vi "ModifyTheValue.vi"(5 "property name":string, 7 "physical channel name":string, 8 "error in (no error)":errorcluster, 9 "Physical Channel Index Cluster":T1, 11 "Data":T2) -> (0 "error out":errorcluster, 2 "Physical Channel Index Cluster Out":T1, 3 "JSON Text Out":string)   [LabVIEW 2018]
uses:
  Ctrl/Data.ctl
  Ctrl/Caps.ctl
  Ctrl/Property.ctl
  Ctrl/PhysicalChannel.ctl
  Ctrl/Register.ctl
  Ctrl/Bitfield.ctl
  Ctrl/Scale.ctl
  Ctrl/ScaleType.ctl
  Ctrl/Enum.ctl
  Ctrl/EnumValue.ctl
  5d60f35e-cdab-4e3f-840e-4fbea60790d1.vi
  29d1ceb7-c941-4ae0-afee-51e252afae0f.vi
  d85de88c-8482-46f7-b9d0-abfa45f3a045.vi
  1afada16-43bf-44c8-a6ff-f358297126fe.vi
  df0b0e95-b0f6-4fc3-aeb6-1b22980748d9.vi
  ef347f2e-25c4-456b-8f90-f769631818f0.vi
  48839aac-ef3d-4912-a59c-d226e3977f89.vi
  0d674d4d-9f77-479f-94dc-be3b3816c1ec.vi
  5f0e6cbb-7cc1-45ab-b940-981c8c673de9.vi
  23bd61ce-0b3e-4435-9956-657a3c4ab8a9.vi
  1678344b-5bca-4df5-9ec5-619e6fe0b93b.vi
  e57232c7-e2d1-4d73-8c4d-58346bc82039.vi
  0e2d7ef8-d2e0-4754-b94e-53af8bd3d5fc.vi
  994b2aef-debc-40fb-8bd7-3405b5177060.vi
  ea1eb992-5890-4c98-ba09-5e0d2d65d542.vi
  <vilib>/JDP Science/JSONtext/String Subset.vi
  <vilib>/JDP Science/JSONtext/Parsing/Parse Full Path or Item Name.vi
  <vilib>/JDP Science/JSONtext/Offset/Find Item Locations by Path.vi
  <vilib>/JDP Science/JSONtext/JSON text to Variant.vi
  <vilib>/JDP Science/JSONtext/Variant to JSON Text.vi
  <vilib>/Utility/Data Type/NI_Data Type.lvlib
  <vilib>/JDP Science/JSONtext/JSONtext.lvlib
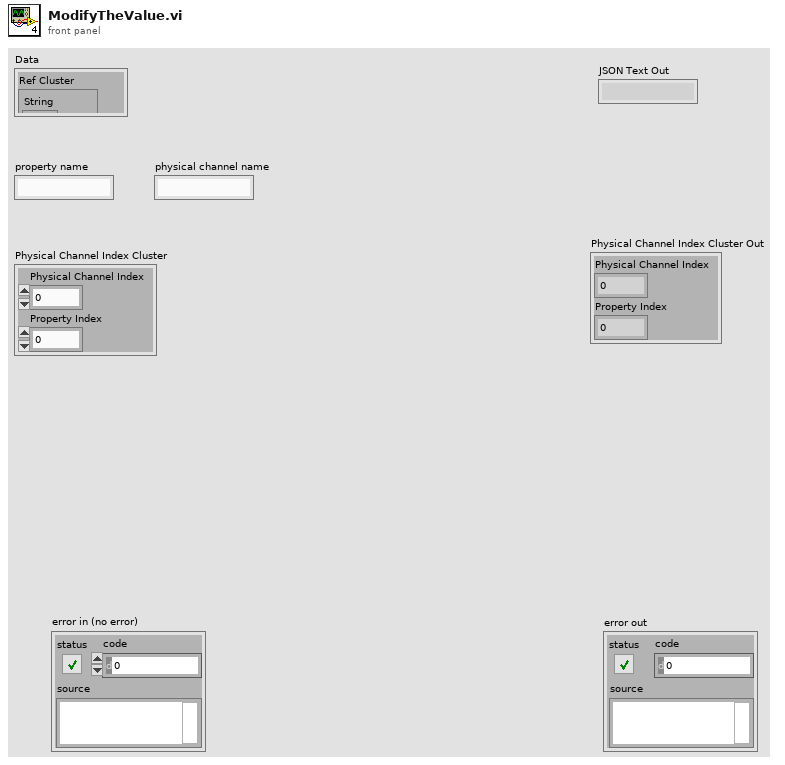
[diagram p1: front panel]
types:
  T1 = cluster{"Physical Channel Index":i32, "Property Index":i32}
  T2 = typedef "Data.ctl" = cluster{"Ref Cluster":cluster{"String":refnum<vi>, "U8":refnum<vi>, "I8":refnum<vi>, "U32":refnum<vi>, "I32":refnum<vi>, "U64":refnum<vi>, "I64":refnum<vi>, "Ring":refnum<vi>, "DBL":refnum<vi>, "Add":refnum<vi>, "Remove":refnum<vi>, "Property tree":refnum<vi>, "confirm":refnum<vi>}, "JSON Text":string, "Original JSON Text":string, "Caps":T3, "SLSC Output Tree":cluster{"Left Cell String":string, "Child Text":string[], "Child Tag":string, "Item Indent":i32, "Child Only?":bool, "Glyph Index":i32, "offline value":variant}[], "Ref Index and Control Type":cluster{"index":i32, "Datatype":string}, "Selected Type and name":cluster{"Selected Type":enum16{"Property", "Physical Channel", "Other"}, "Selected Property Name":string}, "Update whole Tree?":bool}
  T3 = typedef "Caps.ctl" = cluster{"properties":T4[], "physical channels":T5[], "registers":T6[], "scales":T8[], "enums":T10[], "productName":string}
  T4 = typedef "Property.ctl" = cluster{"name":string, "bitfield":string, "value":variant, "dataType":string, "min":variant, "max":variant, "scale":string, "access":string}
  T5 = typedef "PhysicalChannel.ctl" = cluster{"name":string, "properties":T4[]}
  T6 = typedef "Register.ctl" = cluster{"name":string, "address":i32, "size":i32, "bitfields":T7[], "initialValue":variant, "connectedProperties":string[]}
  T7 = typedef "Bitfield.ctl" = cluster{"name":string, "offset":i32, "size":i32, "signed":bool}
  T8 = typedef "Scale.ctl" = cluster{"name":string, "type":T9, "params":variant}
  T9 = typedef "ScaleType.ctl" = enum16{"NoScale", "Table", "Polynomial", "Linear"}
  T10 = typedef "Enum.ctl" = cluster{"name":string, "values":T11[]}
  T11 = typedef "EnumValue.ctl" = cluster{"name":string, "value":i32}
  T12 = typedef "NI_Data Type.lvlib/Data Type.ctl" = enum8{"Invalid Type", "Void", "I8", "I16", "I32", "I64", "U8", "U16", "U32", "U64", "Single Float", "Double Float", "Extended Float", "Single Complex", "Double Complex", "Extended Complex", "Enum U8", "Enum U16", "Enum U32", "Enum U64", "Single Float With Unit", "Double Float With Unit", "Extended Float With Unit", "Single Complex with Unit", "Double Complex with Unit", "Extended Complex with Unit", "Boolean", "String", "Path", "Picture", "Tag", "Array", "Cluster", "Variant", "LV Variant", "Waveform", "Timestamp", "Digital Waveform", "Digital Data", "ExpressData", "Refnum", "External Data", "VI", "Poly VI", "LabVIEW Class Instance", "Fixed Point"}
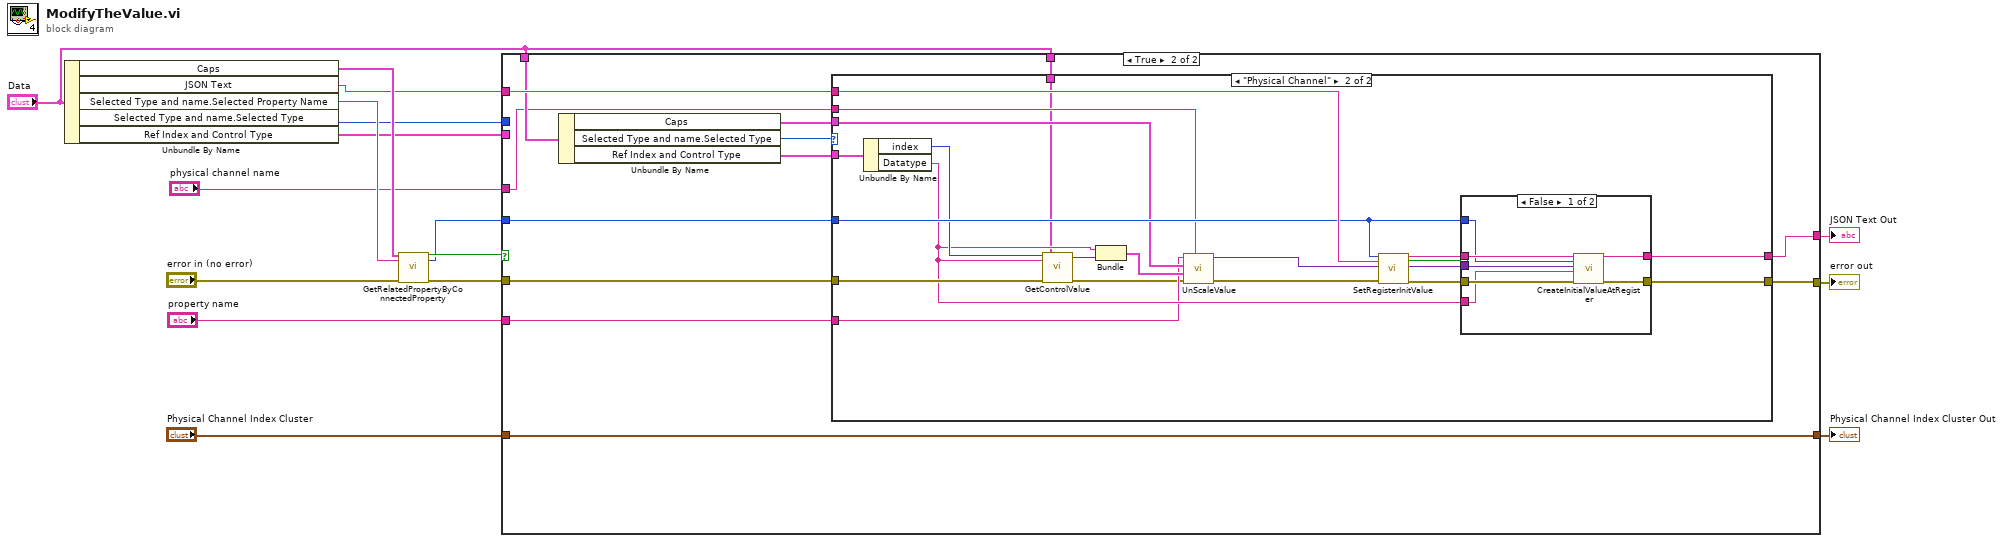
[diagram p0: block diagram]
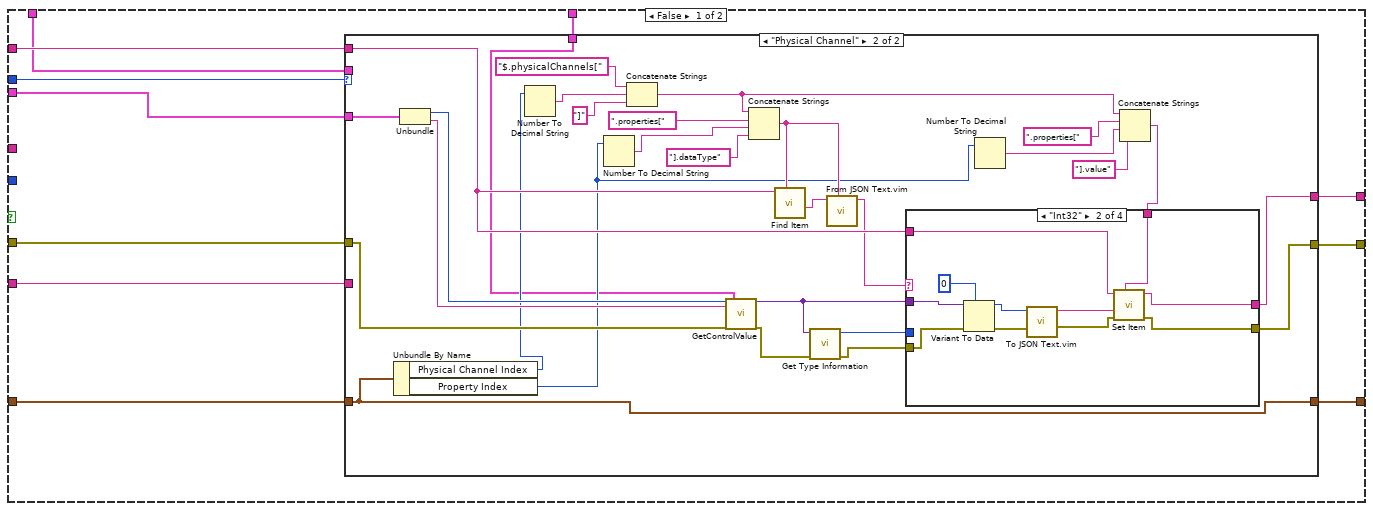
[diagram p2: hidden frame]
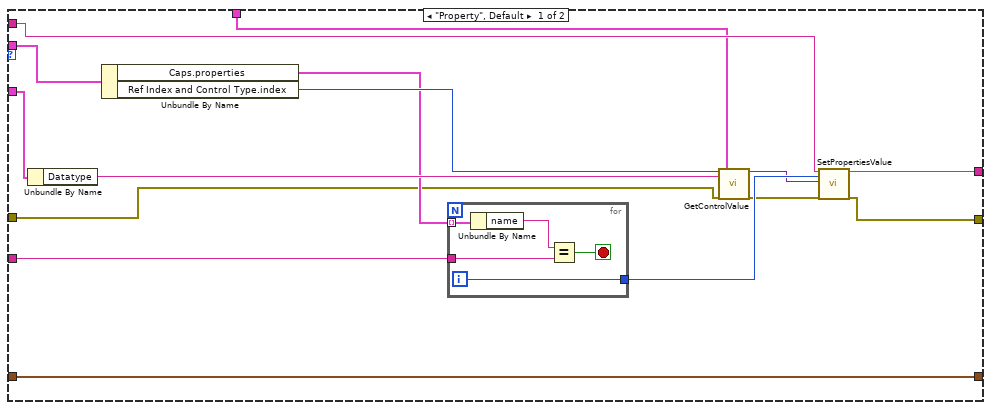
[diagram p3: hidden frame]
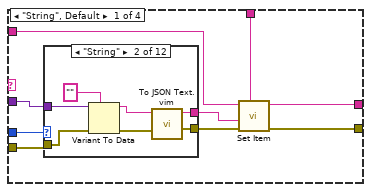
[diagram p4: hidden frame]
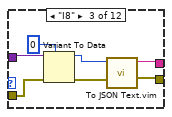
[diagram p6: hidden frame]
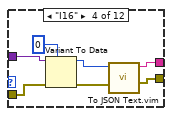
[diagram p7: hidden frame]
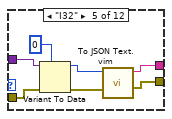
[diagram p8: hidden frame]
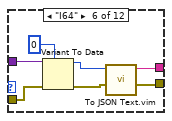
[diagram p9: hidden frame]
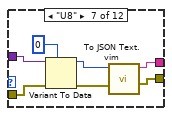
[diagram p10: hidden frame]
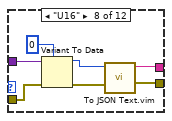
[diagram p11: hidden frame]
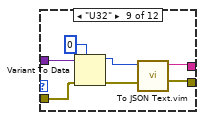
[diagram p12: hidden frame]
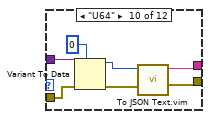
[diagram p13: hidden frame]
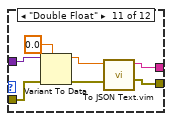
[diagram p14: hidden frame]
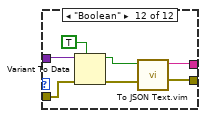
[diagram p15: hidden frame]
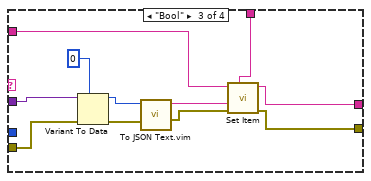
[diagram p16: hidden frame]
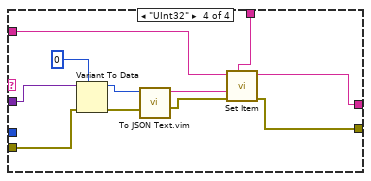
[diagram p17: hidden frame]
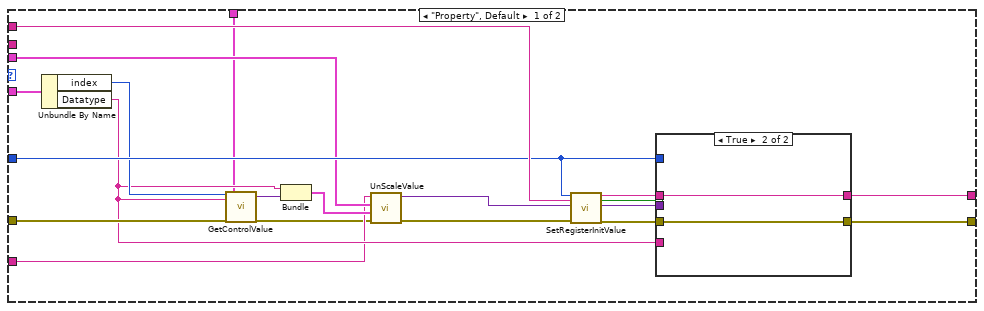
[diagram p18: hidden frame]
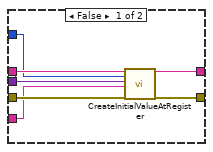
[diagram p19: hidden frame]
diagram:
  n1 = Unbundle By Name("Data") -> ("Caps"=w15:T3, "JSON Text"=w9:string, "Selected Type and name.Selected Property Name"=w14:string, "Selected Type and name.Selected Type"=w8:enum16{"Property", "Physical Channel", "Other"}, "Ref Index and Control Type"=w7:cluster{"index":i32, "Datatype":string})
  n2 = call "GetRelatedPropertyByConnectedProperty.vi"("Caps"=w15, "PropertyName"=w14, "error in (no error)"="error in (no error)") -> ("Find?"=w16:bool, "index of register"=w12:i32, "error out"=w11:errorcluster)  [unwired: 13 in, 1 out]
  n3 = case shown="True" w16 {
    tunnel: "property name" -> [w17 w198]
    tunnel: w11 -> [w26 w202]
    tunnel: w9 -> [w27 w209]
    tunnel: [w25 w208] -> w4
    tunnel: w12 -> [_ w207]
    tunnel: [w24 w206] -> w3
    tunnel: "Data" -> [w23 w205]
    tunnel: "Physical Channel Index Cluster" -> [w22 w200]
    tunnel: [w21 w200] -> w2
    tunnel: "Data" -> [w20 w199]
    tunnel: w8 -> [w19 _]
    tunnel: w7 -> [w18 _]
    tunnel: "physical channel name" -> [_ w197]
    frame False {
      n4 = case shown="\"Physical Channel\"" w19 {
        tunnel: w27 -> [w37 w62]
        tunnel: w26 -> [w35 w75]
        tunnel: [w34 w52] -> w25
        tunnel: [w33 w51] -> w24
        tunnel: w23 -> [w32 _]
        tunnel: w18 -> [w31 w76]
        tunnel: w22 -> [w29 w50]
        tunnel: w17 -> [w30 _]
        tunnel: [w29 w50] -> w21
        tunnel: w20 -> [w28 w48]
        frame "Property", Default {
          n5 = Unbundle By Name(w31) -> ("Datatype"=w42:string)
          n6 = Unbundle By Name(w32) -> ("Caps.properties"=w40:T4[], "Ref Index and Control Type.index"=w41:i32)
          n7 = for {
            tunnel: w40 -> [w47] mode=indexing
            tunnel: w30 -> [w45]
            tunnel: [w43] -> w39
            i -> [w43]
            stop <- w44 stop-if-true
            n8 = Unbundle By Name(w47) -> ("name"=w46:string)
            n9 = Equal?(x=w46, y=w45) -> (x = y?=w44:bool)
          }
          n10 = call "GetControlValue.vi"("index"=w41, "Datatype"=w42, "error in (no error)"=w35, "Data"=w28) -> ("Value"=w38:variant, "error out"=w36:errorcluster)  [unwired: 14 in]
          n11 = call "SetPropertiesValue.vi"("JSON"=w37, "Index"=w39, "Variant"=w38, "error in (no error)"=w36) -> ("<JSON>"=w34:string, "error out"=w33:errorcluster)  [unwired: 14 in]
        }
        frame "Physical Channel" {
          n12 = Unbundle By Name(w50) -> ("Physical Channel Index"=w58:i32, "Property Index"=w54:i32)
          n13 = Unbundle(w76) -> ("index"=w74:i32, "Datatype"=w73:string)
          n14 = Number To Decimal String(number=w58) -> (decimal integer string=w67:string)  [unwired: 1 in]
          n15 = Number To Decimal String(number=w54) -> (decimal integer string=w68:string)  [unwired: 1 in]
          n16 = Concatenate Strings("$.physicalChannels[", w67, "]") -> (w49:string)
          n17 = call "GetControlValue.vi"("index"=w74, "Datatype"=w73, "error in (no error)"=w75, "Data"=w48) -> ("Value"=w69:variant, "error out"=w71:errorcluster)  [unwired: 14 in]
          n18 = Concatenate Strings(w49, ".properties[", w68, "].dataType" ("string")) -> (w55:string)
          n19 = call <vilib>:"Find Item.vi"("$Path or Item Name"=w55, "JSON"=w62) -> ("<JSON>"=w61:string)  [unwired: 6 in, 3 out]
          n20 = call <vilib>:"Get Type Information.vi"("error in (no error)"=w71, "Variant"=w69) -> ("error out"=w70:errorcluster, "Type"=w72:T12)  [unwired: 5 in, 3 out]
          n21 = call "From JSON Text.vim"("Data Type and Default Value"=w55, "JSON"=w61) -> ("Data out"=w60:string)  [unwired: 8 in, 1 out]
          n22 = Number To Decimal String(number=w54) -> (decimal integer string=w57:string)  [unwired: 1 in]
          n23 = Concatenate Strings(w49, ".properties[", w57, "].value" ("string")) -> (w53:string)
          n24 = case shown="\"Int32\"" w60 {
            tunnel: w69 -> [w85 w171 w185 w196]
            tunnel: [w83 w170 w181 w192] -> w52
            tunnel: w72 -> [w82 _ _ _]
            tunnel: w70 -> [w81 w169 w180 w191]
            tunnel: [w79 w166 w177 w188] -> w51
            tunnel: w53 -> [w78 w165 w176 w187]
            tunnel: w62 -> [w77 w164 w175 w186]
            frame "String", Default {
              n25 = case shown="\"String\"" w82 {
                tunnel: w85 -> [_ w93 w99 w106 w113 w120 w127 w134 w141 w148 w155 w161]
                tunnel: [_ w90 w97 w105 w111 w119 w125 w132 w139 w146 w153 w160] -> w84
                tunnel: w81 -> [w86 w89 w96 w103 w110 w117 w124 w131 w138 w145 w152 w159]
                tunnel: [w86 w87 w94 w101 w108 w115 w122 w129 w136 w143 w150 w157] -> w80
                frame "Invalid Type", Default {
                }
                frame "String" {
                  n26 = Variant To Data(error in=w89, type="", Variant=w93) -> (data=w91:string, error out=w88:errorcluster)
                  n27 = call "To JSON Text.vim"("error in (no error)"=w88, "Anything"=w91) -> ("error out"=w87:errorcluster, "<JSON>"=w90:string)  [unwired: 8 in]
                }
                frame "I8" {
                  n28 = Variant To Data(error in=w96, type=i8 0, Variant=w99) -> (data=w100:i8, error out=w95:errorcluster)
                  n29 = call "To JSON Text.vim"("error in (no error)"=w95, "Anything"=w100) -> ("error out"=w94:errorcluster, "<JSON>"=w97:string)  [unwired: 8 in]
                }
                frame "I16" {
                  n30 = Variant To Data(error in=w103, type=i16 0, Variant=w106) -> (data=w107:i16, error out=w102:errorcluster)
                  n31 = call "To JSON Text.vim"("error in (no error)"=w102, "Anything"=w107) -> ("error out"=w101:errorcluster, "<JSON>"=w105:string)  [unwired: 8 in]
                }
                frame "I32" {
                  n32 = Variant To Data(error in=w110, type=0, Variant=w113) -> (data=w114:i32, error out=w109:errorcluster)
                  n33 = call "To JSON Text.vim"("error in (no error)"=w109, "Anything"=w114) -> ("error out"=w108:errorcluster, "<JSON>"=w111:string)  [unwired: 8 in]
                }
                frame "I64" {
                  n34 = Variant To Data(error in=w117, type=i64 0, Variant=w120) -> (data=w121:i64, error out=w116:errorcluster)
                  n35 = call "To JSON Text.vim"("error in (no error)"=w116, "Anything"=w121) -> ("error out"=w115:errorcluster, "<JSON>"=w119:string)  [unwired: 8 in]
                }
                frame "U8" {
                  n36 = Variant To Data(error in=w124, type=u8 0, Variant=w127) -> (data=w128:u8, error out=w123:errorcluster)
                  n37 = call "To JSON Text.vim"("error in (no error)"=w123, "Anything"=w128) -> ("error out"=w122:errorcluster, "<JSON>"=w125:string)  [unwired: 8 in]
                }
                frame "U16" {
                  n38 = Variant To Data(error in=w131, type=u16 0, Variant=w134) -> (data=w135:u16, error out=w130:errorcluster)
                  n39 = call "To JSON Text.vim"("error in (no error)"=w130, "Anything"=w135) -> ("error out"=w129:errorcluster, "<JSON>"=w132:string)  [unwired: 8 in]
                }
                frame "U32" {
                  n40 = Variant To Data(error in=w138, type=u32 0, Variant=w141) -> (data=w142:u32, error out=w137:errorcluster)
                  n41 = call "To JSON Text.vim"("error in (no error)"=w137, "Anything"=w142) -> ("error out"=w136:errorcluster, "<JSON>"=w139:string)  [unwired: 8 in]
                }
                frame "U64" {
                  n42 = Variant To Data(error in=w145, type=u64 0, Variant=w148) -> (data=w149:u64, error out=w144:errorcluster)
                  n43 = call "To JSON Text.vim"("error in (no error)"=w144, "Anything"=w149) -> ("error out"=w143:errorcluster, "<JSON>"=w146:string)  [unwired: 8 in]
                }
                frame "Double Float" {
                  n44 = Variant To Data(error in=w152, type=0.0, Variant=w155) -> (data=w156:dbl, error out=w151:errorcluster)
                  n45 = call "To JSON Text.vim"("error in (no error)"=w151, "Anything"=w156) -> ("error out"=w150:errorcluster, "<JSON>"=w153:string)  [unwired: 8 in]
                }
                frame "Boolean" {
                  n46 = Variant To Data(error in=w159, type=TRUE, Variant=w161) -> (data=w163:bool, error out=w158:errorcluster)
                  n47 = call "To JSON Text.vim"("error in (no error)"=w158, "Anything"=w163) -> ("error out"=w157:errorcluster, "<JSON>"=w160:string)  [unwired: 8 in]
                }
              }
              n48 = call <vilib>:"Set Item.vi"("$Path or Item Name"=w78, "error in (no error)"=w80, "JSON to Insert"=w84, "JSON"=w77) -> ("error out"=w79:errorcluster, "<JSON>"=w83:string)  [unwired: 4 in, 1 out]
            }
            frame "Int32" {
              n49 = Variant To Data(error in=w169, type=0, Variant=w171) -> (data=w173:i32, error out=w168:errorcluster)
              n50 = call "To JSON Text.vim"("error in (no error)"=w168, "Anything"=w173) -> ("error out"=w167:errorcluster, "<JSON>"=w172:string)  [unwired: 8 in]
              n51 = call <vilib>:"Set Item.vi"("$Path or Item Name"=w165, "error in (no error)"=w167, "JSON to Insert"=w172, "JSON"=w164) -> ("error out"=w166:errorcluster, "<JSON>"=w170:string)  [unwired: 4 in, 1 out]
            }
            frame "Bool" {
              n52 = Variant To Data(error in=w180, type=u16 0, Variant=w185) -> (data=w183:u16, error out=w179:errorcluster)
              n53 = call "To JSON Text.vim"("error in (no error)"=w179, "Anything"=w183) -> ("error out"=w178:errorcluster, "<JSON>"=w182:string)  [unwired: 8 in]
              n54 = call <vilib>:"Set Item.vi"("$Path or Item Name"=w176, "error in (no error)"=w178, "JSON to Insert"=w182, "JSON"=w175) -> ("error out"=w177:errorcluster, "<JSON>"=w181:string)  [unwired: 4 in, 1 out]
            }
            frame "UInt32" {
              n55 = Variant To Data(error in=w191, type=u32 0, Variant=w196) -> (data=w194:u32, error out=w190:errorcluster)
              n56 = call "To JSON Text.vim"("error in (no error)"=w190, "Anything"=w194) -> ("error out"=w189:errorcluster, "<JSON>"=w193:string)  [unwired: 8 in]
              n57 = call <vilib>:"Set Item.vi"("$Path or Item Name"=w187, "error in (no error)"=w189, "JSON to Insert"=w193, "JSON"=w186) -> ("error out"=w188:errorcluster, "<JSON>"=w192:string)  [unwired: 4 in, 1 out]
            }
          }
        }
      }
    }
    frame True {
      n58 = Unbundle By Name(w205) -> ("Caps"=w201:T3, "Selected Type and name.Selected Type"=w204:enum16{"Property", "Physical Channel", "Other"}, "Ref Index and Control Type"=w203:cluster{"index":i32, "Datatype":string})
      n59 = case shown="\"Physical Channel\"" w204 {
        tunnel: w209 -> [w228 w258]
        tunnel: [w224 w254] -> w208
        tunnel: w207 -> [w222 w252]
        tunnel: [w220 w250] -> w206
        tunnel: w203 -> [w219 w249]
        tunnel: w202 -> [w217 w247]
        tunnel: w201 -> [w214 w244]
        tunnel: w198 -> [w212 w242]
        tunnel: w197 -> [_ w241]
        tunnel: w199 -> [w211 w240]
        frame "Property", Default {
          n60 = Unbundle By Name(w219) -> ("index"=w218:i32, "Datatype"=w213:string)
          n61 = call "GetControlValue.vi"("index"=w218, "Datatype"=w213, "error in (no error)"=w217, "Data"=w211) -> ("Value"=w216:variant, "error out"=w210:errorcluster)  [unwired: 14 in]
          n62 = Bundle("Datatype"=w213, "Value"=w216) -> (w215:cluster{"Datatype":string, "Value":variant})  [unwired: 1 in]
          n63 = call "UnScaleValue.vi"("error in (no error)"=w210, "Type&Value"=w215, "Caps"=w214, "property"=w212) -> ("error out"=w227:errorcluster, "Variant"=w229:variant)  [unwired: 6 in]
          n64 = call "SetRegisterInitValue.vi"("Index"=w222, "JSON"=w228, "Variant"=w229, "error in (no error)"=w227) -> ("<JSON>"=w225:string, "Replaced"=w226:bool, "Variant output"=w223:variant, "error out"=w221:errorcluster)  [unwired: 12 in]
          n65 = case shown="True" w226 {
            tunnel: w225 -> [w236 w237]
            tunnel: [w235 w237] -> w224
            tunnel: w223 -> [w233 _]
            tunnel: w222 -> [w234 _]
            tunnel: w213 -> [w230 _]
            tunnel: w221 -> [w232 w238]
            tunnel: [w231 w238] -> w220
            frame False {
              n66 = call "CreateInitialValueAtRegister.vi"("JSON"=w236, "Register Index"=w234, "Value"=w233, "DataType"=w230, "error in (no error)"=w232) -> ("<JSON>"=w235:string, "error out"=w231:errorcluster)  [unwired: 13 in]
            }
            frame True {
            }
          }
        }
        frame "Physical Channel" {
          n67 = Unbundle By Name(w249) -> ("index"=w248:i32, "Datatype"=w243:string)
          n68 = call "GetControlValue.vi"("index"=w248, "Datatype"=w243, "error in (no error)"=w247, "Data"=w240) -> ("Value"=w246:variant, "error out"=w239:errorcluster)  [unwired: 14 in]
          n69 = Bundle("Datatype"=w243, "Value"=w246) -> (w245:cluster{"Datatype":string, "Value":variant})  [unwired: 1 in]
          n70 = call "UnScaleValue.vi"("physical channel"=w241, "error in (no error)"=w239, "Type&Value"=w245, "Caps"=w244, "property"=w242) -> ("error out"=w257:errorcluster, "Variant"=w259:variant)  [unwired: 5 in]
          n71 = call "SetRegisterInitValue.vi"("Index"=w252, "JSON"=w258, "Variant"=w259, "error in (no error)"=w257) -> ("<JSON>"=w255:string, "Replaced"=w256:bool, "Variant output"=w253:variant, "error out"=w251:errorcluster)  [unwired: 12 in]
          n72 = case shown="False" w256 {
            tunnel: w255 -> [w266 w267]
            tunnel: [w265 w267] -> w254
            tunnel: w253 -> [w263 _]
            tunnel: w252 -> [w264 _]
            tunnel: w243 -> [w260 _]
            tunnel: w251 -> [w262 w268]
            tunnel: [w261 w268] -> w250
            frame False {
              n73 = call "CreateInitialValueAtRegister.vi"("JSON"=w266, "Register Index"=w264, "Value"=w263, "DataType"=w260, "error in (no error)"=w262) -> ("<JSON>"=w265:string, "error out"=w261:errorcluster)  [unwired: 13 in]
            }
            frame True {
            }
          }
        }
      }
    }
  }
  "JSON Text Out" <- w4
  "error out" <- w3
  "Physical Channel Index Cluster Out" <- w2
